vi "Read lifter config_Calibration info.vi"(4 "error in (no error)":errorcluster) -> (0 "error out":errorcluster, 2 "Insert":string, 3 "Date":string)   [LabVIEW 2019]
uses:
  <vilib>/Utility/config.llb/Read Key (String).vi
  <vilib>/Utility/config.llb/NI_LVConfig.lvlib
panel:
  out "appended path":path
  out "concatenated string":string
  in  "File Name":string="Lifter config"
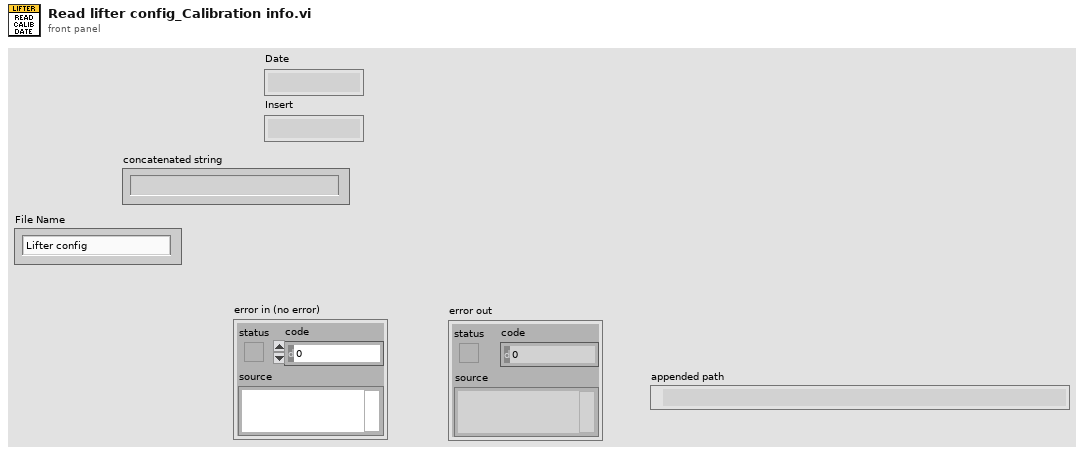
[diagram p1: front panel]
types:
  T1 = typedef "NI_LVConfig.lvlib/Config Data RefNum.ctl" = refnum<k1>
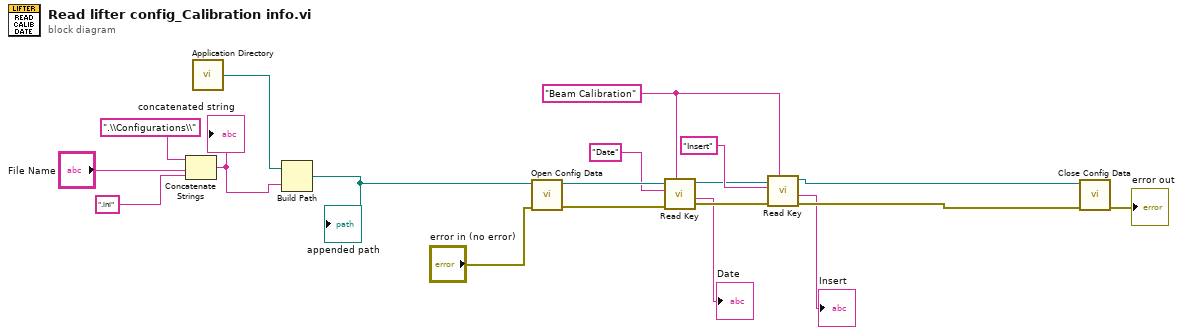
[diagram p0: block diagram]
diagram:
  w7 = "Beam Calibration" ("section")
  n1 = Concatenate Strings(".\\Configurations\\" ("string"), "File Name", ".ini" ("string")) -> (w17:string)
  "concatenated string" <- w17
  n2 = call <vilib>:"Application Directory.vi"() -> ("Application Directory"=w15:path)
  n3 = Build Path(base path=w15, name or relative path=w17) -> (appended path=w12:path)
  "appended path" <- w12
  n4 = call <vilib>:"Open Config Data.vi"("error in (no error)"="error in (no error)", "configuration file path"=w12) -> ("error out"=w10:errorcluster, "refnum"=w11:T1)  [unwired: 7 in, 1 out]
  n5 = call-poly <vilib>:"Read Key.vi"("section"=w7, "error in (no error)"=w10, "key"="Date" ("section"), "refnum"=w11) -> ("error out"=w4:errorcluster, "value"=→"Date":string, "refnum out"=w3:T1)  [unwired: 4 in, 1 out]
  n6 = call-poly <vilib>:"Read Key.vi"("section"=w7, "error in (no error)"=w4, "key"="Insert" ("section"), "refnum"=w3) -> ("error out"=w5:errorcluster, "value"=→"Insert":string, "refnum out"=w6:T1)  [unwired: 4 in, 1 out]
  n7 = call <vilib>:"Close Config Data.vi"("error in (no error)"=w5, "refnum"=w6) -> ("error out"=→"error out":errorcluster)  [unwired: 8 in, 1 out]
